vi "draw_scale_bar.vi"(5 "precision":i16=2, 7 "fraction of image dimension":dbl=0.1, 8 "error in (no error)":errorcluster, 10 "angle":dbl[unit], 11 "Image in":refnum<class "Image.lvclass">=refnum) -> (0 "error out":errorcluster, 3 "Image out":refnum<class "Image.lvclass">)   [LabVIEW 2010, in "Image.lvclass"]
uses:
  Image.lvclass
  <vilib>/vision/Image Controls.llb/IMAQ Image.ctl
  Image.lvclass/Image.ctl
  ErrorController/ErrorController/class_data.vi
  ErrorController/ErrorController/ErrorController.lvclass
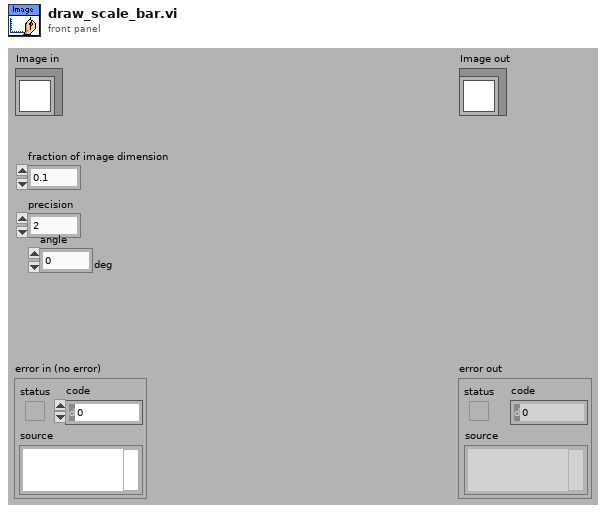
[diagram p1: front panel]
types:
  T1 = cluster{"Desired Font (Application)":enum16{"User-specified Font", "Application Font", "System Font", "Dialog Font"}, "[User-specified Font]":cluster{"Font Name":string, "Size":i16, "Strikeout?":bool, "Italic?":bool, "Underline?":bool, "Outline?":bool, "Shadow?":bool, "Bold?":bool, "Rotation Angle":dbl}, "Horizontal Alignment":i16, "Vertical Alignment":i16}
  T2 = typedef "IMAQ Image.ctl" = refnum<image>
  T3 = typedef "Image.lvclass/unit.ctl" = enum16{"um", "s"}
  T4 = cluster{"Desired Font (Application)":enum16{"User-specified Font", "Application Font", "System Font", "Dialog Font"}, "[User-specified Font]":cluster{"Font Name":string, "Size":i16, "Strikeout?":bool, "Italic?":bool, "Underline?":bool, "Outline?":bool, "Shadow?":bool, "Bold?":bool, "Rotation Angle":dbl}, "Horizontal Alignment":i16, "Vertical Alignment":i16}[]
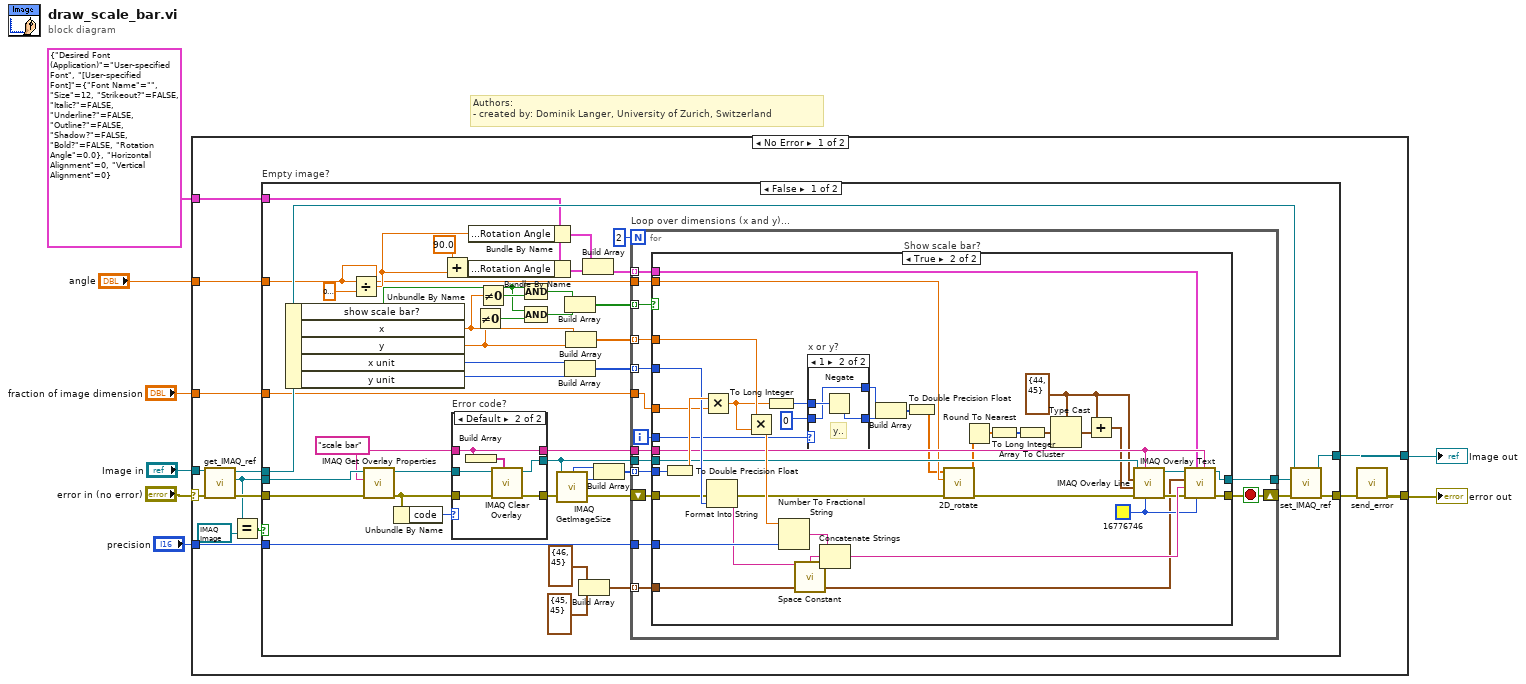
[diagram p0: block diagram]
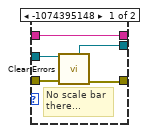
[diagram p4: hidden frame]
diagram:
  # "Authors: \n- created by: Dominik Langer, University of Zurich, Switzerland"
  n1 = case shown="No Error" "error in (no error)" {
    selector: "error in (no error)" -> [w22 w142]
    tunnel: [w10 w142] -> w7
    tunnel: [w20 w141] -> w5
    tunnel: "Image in" -> [w21 w141]
    tunnel: T1 {"Desired Font (Application)"=enum."User-specified Font", "[User-specified Font]"={"Font Name"="", "Size"=12, "Strikeout?"=FALSE, "Italic?"=FALSE, "Underline?"=FALSE, "Outline?"=FALSE, "Shadow?"=FALSE, "Bold?"=FALSE, "Rotation Angle"=0.0}, "Horizontal Alignment"=0, "Vertical Alignment"=0} ("Font, Size & Style") -> [w15 _]
    tunnel: "precision" -> [w17 _]
    tunnel: "fraction of image dimension" -> [w16 _]
    tunnel: "angle" -> [w14 _]
    frame No Error {
      n2 = call-dynamic "get_IMAQ_ref.vi"("error in (no error)"=w22, "Image.lvclass in"=w21) -> ("error out"=w18:errorcluster, "Image"=w13:T2, "Image.lvclass out"=w19:refnum<class "Image.lvclass">)  [unwired: 7 out]
      n3 = Equal?(x=w13, y=T2 refnum) -> (x = y?=w12:bool)
      n4 = case "Empty image?" shown="False" w12 {
        tunnel: [w66 w140] -> w9
        tunnel: [w65 w139] -> w20
        tunnel: w19 -> [w64 w139]
        tunnel: w18 -> [w62 w140]
        tunnel: w13 -> [w61 _]
        tunnel: w17 -> [w31 _]
        tunnel: w16 -> [w30 _]
        tunnel: w15 -> [w27 _]
        tunnel: w14 -> [w23 _]
        frame False {
          w59 = "scale bar" ("String")
          n5 = Unbundle By Name(w64) -> ("show scale bar?"=w52:bool, "x"=w47:dbl, "y"=w46:dbl, "x unit"=w45:T3, "y unit"=w44:T3)
          n6 = Divide(x=w23, y=dbl[unit] 0.017453292519943295) -> (x/y=w24:dbl)
          n7 = call "IMAQ Get Overlay Properties"("error in (no error)"=w62, "Group"=w59, "Image"=w61) -> ("error out"=w58:errorcluster, "Image Out"=w60:T2)  [unwired: 5 out]
          n8 = Unbundle By Name(w58) -> ("code"=w57:i32)
          n9 = Add(x=90.0 ("[User-specified Font].Rotation Angle"), y=w24) -> (x+y=w28:dbl)
          n10 = case "Error code?" shown="Default" w57 {
            tunnel: [w130 w138] -> w42
            tunnel: [w129 w137] -> w40
            tunnel: w60 -> [w129 w136]
            tunnel: w59 -> [w132 w133]
            tunnel: w58 -> [w131 w134]
            tunnel: [w132 w133] -> w56
            frame -1074395148 {
              # "No scale bar there..."
              n11 = call <vilib>:"Clear Errors.vi"("error in (no error)"=w131) -> ("error out"=w130:errorcluster)  [unwired: 6 out]
            }
            frame Default {
              n12 = Build Array(w133) -> (w135:string[])
              n13 = call "IMAQ Clear Overlay"("Groups"=w135, "error in (no error)"=w134, "Image"=w136) -> ("error out"=w138:errorcluster, "Image Out"=w137:T2)  [unwired: 7 out]
            }
          }
          n14 = Bundle By Name(cluster=w27, "[User-specified Font].Rotation Angle"=w24) -> (w26:T1)
          n15 = Bundle By Name(cluster=w27, "[User-specified Font].Rotation Angle"=w28) -> (w35:T1)
          n16 = Not Equal To 0?(x=w46) -> (x != 0?=w53:bool)
          n17 = Not Equal To 0?(x=w47) -> (x != 0?=w54:bool)
          n18 = Compound Arithmetic op=AND(w52, w54) -> (w50:bool)
          n19 = Compound Arithmetic op=AND(w52, w53) -> (w51:bool)
          n20 = call "IMAQ GetImageSize"("Image"=w40, "error in (no error)"=w42) -> ("Y Resolution"=w38:i32, "X Resolution"=w39:i32, "error out"=w41:errorcluster)  [unwired: 2 out]
          n21 = Build Array(w50, w51) -> (w49:bool[])
          n22 = Build Array(w45, w44) -> (w43:T3[])
          n23 = Build Array(w47, w46) -> (w48:dbl[])
          n24 = Build Array(cluster{"X":i32, "Y":i32} {"X"=46, "Y"=45} ("Origin"), cluster{"X":i32, "Y":i32} {"X"=45, "Y"=45} ("Origin")) -> (w32:cluster{"X":i32, "Y":i32}[])
          n25 = Build Array(w26, w35) -> (w36:T4)
          n26 = Build Array(w39, w38) -> (w37:i32[])
          n27 = for "Loop over dimensions (x and y)..." {
            N: 2 -> [_]
            tunnel: w40 -> [w81]
            tunnel: [w80] -> w63
            tunnel: w56 -> [w79]
            tunnel: w49 -> [w78] mode=indexing
            tunnel: w48 -> [w77] mode=indexing
            tunnel: w43 -> [w76] mode=indexing
            tunnel: w36 -> [w75] mode=indexing
            tunnel: w30 -> [w74]
            shift-right: [w68] -> w67
            shift-left: w41 -> [w82]
            tunnel: w37 -> [w73] mode=indexing
            tunnel: w32 -> [w71] mode=indexing
            tunnel: w31 -> [w70]
            tunnel: w23 -> [w69]
            i -> [w72]
            stop <- w68 stop-if-true
            n28 = case "Show scale bar?" shown="True" w78 {
              tunnel: w82 -> [w84 w105]
              tunnel: [w84 w116] -> w68
              tunnel: w81 -> [w83 w111]
              tunnel: w77 -> [_ w104]
              tunnel: [w83 w110] -> w80
              tunnel: w79 -> [_ w112]
              tunnel: w76 -> [_ w118]
              tunnel: w75 -> [_ w108]
              tunnel: w74 -> [_ w107]
              tunnel: w73 -> [_ w106]
              tunnel: w72 -> [_ w102]
              tunnel: w71 -> [_ w101]
              tunnel: w70 -> [_ w100]
              tunnel: w69 -> [_ w94]
              frame False {
              }
              frame True {
                w85 = cluster{"X":i32, "Y":i32} {"X"=44, "Y"=45} ("Start Point")
                w114 = u32 16776746 ("Color")
                n29 = To Double Precision Float(number=w106) -> (double precision float=w121:dbl)
                n30 = Multiply(x=w121, y=w107) -> (x*y=w103:dbl)
                n31 = Format Into String(error in=w105, w118) -> (resulting string=w99:string, error out=w88:errorcluster)  [unwired: 2 in]
                n32 = Multiply(x=w104, y=w103) -> (x*y=w117:dbl)
                n33 = To Long Integer(number=w103) -> (32bit integer=w123:i32)
                n34 = Number To Fractional String(number=w117, precision (6)=w100) -> (F-format string=w120:string)  [unwired: 2 out]
                n35 = call <vilib>:"Space Constant.vi"() -> ("String"=w98:string)
                n36 = case "x or y?" shown="1" w102 {
                  tunnel: w123 -> [w125 w128]
                  tunnel: 0 ("Y") -> [w124 w126]
                  tunnel: [w125 w126] -> w97
                  tunnel: [w124 w127] -> w96
                  frame 0, Default {
                    # "x..."
                  }
                  frame 1 {
                    # "y.."
                    n37 = Negate(x=w128) -> (-x=w127:i32)
                  }
                }
                n38 = Concatenate Strings(w120, w98, w99) -> (w119:string)
                n39 = Build Array(w97, w96) -> (w95:i32[])
                n40 = To Double Precision Float(number=w95) -> (double precision float=w93:dbl[])
                n41 = call "2D_rotate.vi"("error in (no error)"=w88, "angle"=w94, "input vector"=w93) -> ("error out"=w87:errorcluster, "output vector"=w92:dbl[])  [unwired: 7 in]
                n42 = Round To Nearest(number=w92) -> (nearest integer value=w91:dbl[])
                n43 = To Long Integer(number=w91) -> (32bit integer=w90:i32[])
                n44 = Array To Cluster(array=w90) -> (cluster=w89:cluster{"[0]":i32, "[1]":i32})
                n45 = Type Cast(type=w85, x=w89) -> (*(type *) &x=w86:cluster{"X":i32, "Y":i32})
                n46 = Add(x=w85, y=w86) -> (x+y=w109:cluster{"X":i32, "Y":i32})
                n47 = call "IMAQ Overlay Line"("Color"=w114, "Group"=w112, "error in (no error)"=w87, "End Point"=w109, "Start Point"=w85, "Image"=w111) -> ("error out"=w115:errorcluster, "Image Out"=w113:T2)  [unwired: 4 out]
                n48 = call "IMAQ Overlay Text"("Group"=w112, "Text Color (black)"=w114, "Font, Size & Style"=w108, "error in (no error)"=w115, "String"=w119, "Origin"=w101, "Image"=w113) -> ("error out"=w116:errorcluster, "Image Out"=w110:T2)  [unwired: 1 in, 2 out]
              }
            }
          }
          n49 = call-dynamic "set_IMAQ_ref.vi"("error in (no error)"=w67, "Image"=w63, "Image.lvclass in"=w64) -> ("error out"=w66:errorcluster, "Image.lvclass out"=w65:refnum<class "Image.lvclass">)  [unwired: 7 out]
        }
        frame True {
        }
      }
      n50 = call "send_error.vi"("error in (no error)"=w9) -> ("error out"=w10:errorcluster)  [unwired: 10 in]
    }
    frame Error {
    }
  }
  "error out" <- w7
  "Image out" <- w5
